vi "calc rect to polar.vi"(10 "XY":cluster{"X":dbl, "Y":dbl}) -> (1 "angle (rad)":dbl, 2 "angle (deg)":dbl, 3 "Magnitude":dbl)   [LabVIEW 2023]
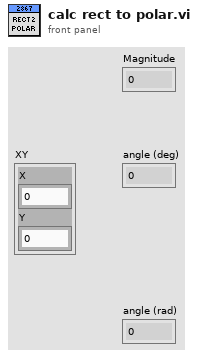
[diagram p1: front panel]
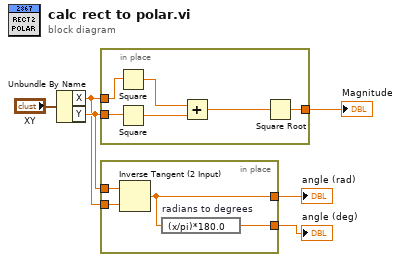
[diagram p0: block diagram]
diagram:
  n1 = Unbundle By Name("XY") -> ("X"=w1:dbl, "Y"=w2:dbl)
  n2 = in-place {
    in-place-border: [w12] -> w6
    in-place-border: w2 -> [w11]
    in-place-border: w1 -> [w10]
    n3 = Square(x=w10) -> (x^2=w8:dbl)
    n4 = Square(x=w11) -> (x^2=w9:dbl)
    n5 = Add(x=w8, y=w9) -> (x+y=w7:dbl)
    n6 = Square Root(x=w7) -> (sqrt(x)=w12:dbl)
  }
  "Magnitude" <- w6
  n7 = in-place {
    in-place-border: [w16] -> w4
    in-place-border: [w15] -> w3
    in-place-border: w2 -> [w14]
    in-place-border: w1 -> [w13]
    n8 = Inverse Tangent (2 Input)(1:w13, 2:w14) -> (0:w16:dbl)
    n9 = expression code="(x/pi)*180.0" "radians to degrees"(w16) -> (w15:dbl)
  }
  "angle (deg)" <- w3
  "angle (rad)" <- w4
